vi "Test_PXF4_x2.vi"() -> ()   [LabVIEW 2019]
uses:
  <vilib>/NI/Modbus Library/API/Master/Modbus Master.lvclass
panel:
  in  "SV2_set":dbl=70.5 format="%.1f"
  in  "set_SV2":bool
  out "Out_2":bool
  out "SV2":dbl format="%.1f"
  out "PV2":dbl format="%.1f"
  in  "UID2":u8=2
  out "Out_1":bool
  in  "hysteresis_set":i16=1
  in  "set_hyst":bool
  out "time":timestamp format="%<%H:%M:%S\n%Y/%m/%d>T"
  out "hysteresis_get":u16
  in  "get_hyst":bool
  in  "set_SV":bool
  in  "interval":i32=1000
  in  "stop":bool
  out "SV1":dbl format="%.1f"
  out "PV1":dbl format="%.1f"
  in  "SV_set":dbl=70.5 format="%.1f"
  out "error out":errorcluster
  in  "UID1":u8=1
  in  "VISA":refnum<visa-resource-name>="COM7"
  # "CH 1"
  # "CH 2"
  # "°F"
  # "°F"
  # "°F"
  # "°F"
  # "°F"
  # "°F"
  # "°F"
  # "°F"
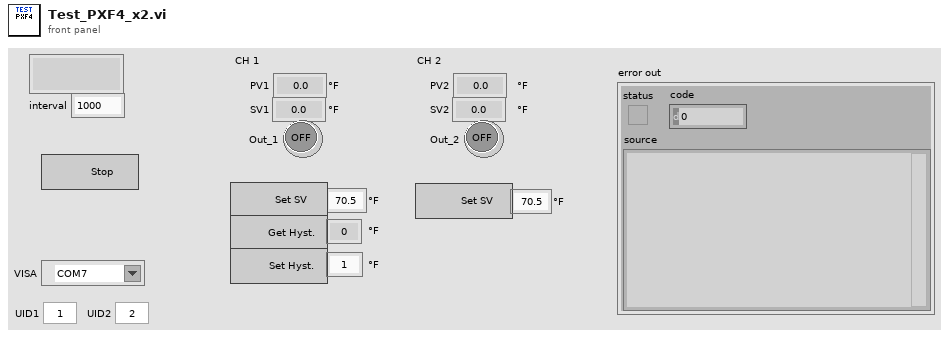
[diagram p1: front panel]
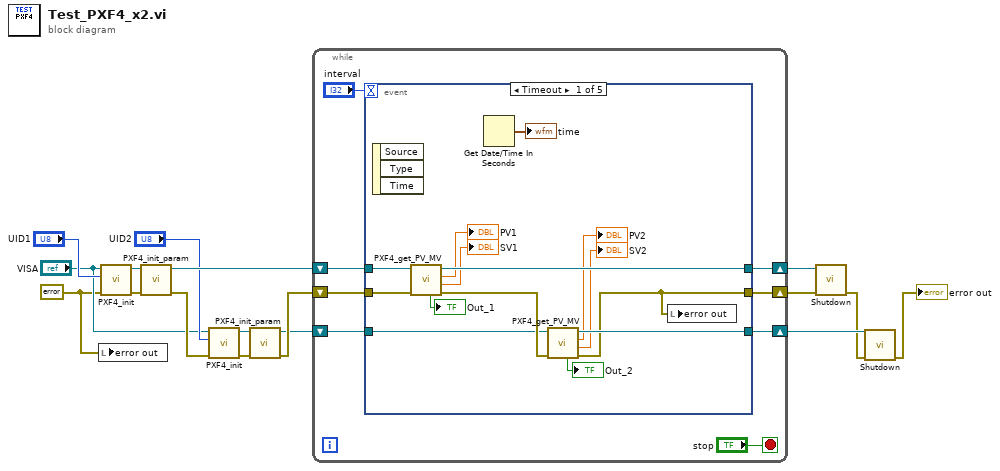
[diagram p0: block diagram]
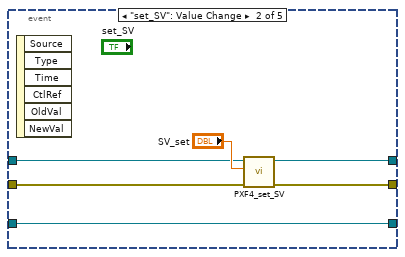
[diagram p2: hidden frame]
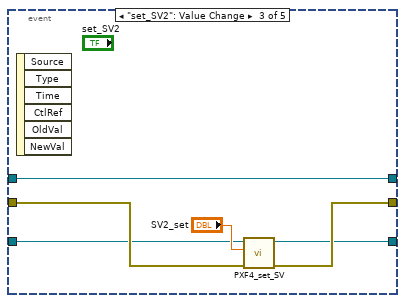
[diagram p3: hidden frame]
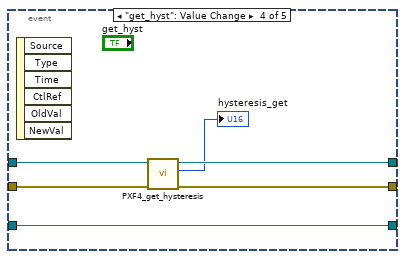
[diagram p4: hidden frame]
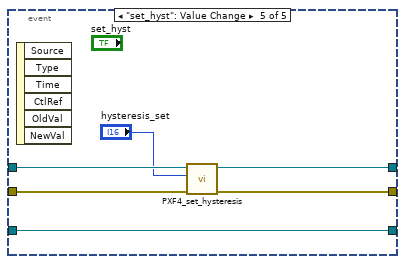
[diagram p5: hidden frame]
diagram:
  w1 = errorcluster {"status"=FALSE, "code"=0, "source"=""} ("error in")
  n1 = local write "error out"(w1) -> ()
  n2 = call "PXF4_init.vi"("error in"=w1, "unit_ID"="UID1", "VISA Refnum in"="VISA") -> ("error out"=w15:errorcluster, "Modbus Master out"=w16:refnum<class "Modbus Master.lvclass">)  [unwired: 7 in]
  n3 = call "PXF4_init_param.vi"("error in"=w15, "Modbus Master in"=w16) -> ("error out"=w9:errorcluster, "Modbus Master out"=w14:refnum<class "Modbus Master.lvclass">)  [unwired: 8 in]
  n4 = call "PXF4_init.vi"("error in"=w9, "unit_ID"="UID2", "VISA Refnum in"="VISA") -> ("error out"=w8:errorcluster, "Modbus Master out"=w11:refnum<class "Modbus Master.lvclass">)  [unwired: 7 in]
  n5 = call "PXF4_init_param.vi"("error in"=w8, "Modbus Master in"=w11) -> ("error out"=w7:errorcluster, "Modbus Master out"=w6:refnum<class "Modbus Master.lvclass">)  [unwired: 8 in]
  n6 = while {
    shift-right: [w22] -> w13
    shift-left: w14 -> [w25]
    shift-right: [w23] -> w12
    shift-left: w7 -> [w24]
    shift-right: [w18] -> w5
    shift-left: w6 -> [w19]
    stop <- "stop" stop-if-true
    n7 = event shown="[0] Timeout" {
      selector: _ -> [_ _ _ _ _]
      dyn-events: _ -> [_ _ _ _ _]
      timeout: "interval" -> [_ _ _ _ _]
      tunnel: w25 -> [w39 w41 w46 w57 w63]
      tunnel: w24 -> [w37 w42 w49 w56 w60]
      tunnel: [w26 w43 w50 w55 w61] -> w23
      tunnel: [w38 w44 w46 w54 w62] -> w22
      tunnel: w19 -> [w31 w40 w48 w52 w58]
      tunnel: [w30 w40 w47 w52 w58] -> w18
      event Timeout {
        n8 = event-data() -> ()  [unwired: 1 in, 3 out]
        n9 = call "PXF4_get_PV_MV.vi"("error in"=w37, "Modbus Master in"=w39) -> ("error out"=w32:errorcluster, "SV"=→"SV1":dbl, "PV"=→"PV1":dbl, "Modbus Master out"=w38:refnum<class "Modbus Master.lvclass">, "Output"=→"Out_1":bool)  [unwired: 5 in]
        n10 = Get Date/Time In Seconds() -> (seconds since 1Jan1904=→"time":timestamp)
        n11 = call "PXF4_get_PV_MV.vi"("error in"=w32, "Modbus Master in"=w31) -> ("error out"=w26:errorcluster, "SV"=→"SV2":dbl, "PV"=→"PV2":dbl, "Modbus Master out"=w30:refnum<class "Modbus Master.lvclass">, "Output"=→"Out_2":bool)  [unwired: 5 in]
        n12 = local write "error out"(w26) -> ()
      }
      event "set_SV": Value Change {
        n13 = event-data() -> ()  [unwired: 1 in, 6 out]
        n14 = call "PXF4_set_SV.vi"("error in"=w42, "SV"="SV_set", "Modbus Master in"=w41) -> ("error out"=w43:errorcluster, "Modbus Master out"=w44:refnum<class "Modbus Master.lvclass">)  [unwired: 7 in]
      }
      event "set_SV2": Value Change {
        n15 = event-data() -> ()  [unwired: 1 in, 6 out]
        n16 = call "PXF4_set_SV.vi"("error in"=w49, "SV"="SV2_set", "Modbus Master in"=w48) -> ("error out"=w50:errorcluster, "Modbus Master out"=w47:refnum<class "Modbus Master.lvclass">)  [unwired: 7 in]
      }
      event "get_hyst": Value Change {
        n17 = event-data() -> ()  [unwired: 1 in, 6 out]
        n18 = call "PXF4_get_hysteresis.vi"("error in"=w56, "Modbus Master in"=w57) -> ("error out"=w55:errorcluster, "hysteresis"=→"hysteresis_get":i16, "Modbus Master out"=w54:refnum<class "Modbus Master.lvclass">)  [unwired: 7 in]
      }
      event "set_hyst": Value Change {
        n19 = event-data() -> ()  [unwired: 1 in, 6 out]
        n20 = call "PXF4_set_hysteresis.vi"("error in"=w60, "hysteresis"="hysteresis_set", "Modbus Master in"=w63) -> ("error out"=w61:errorcluster, "Modbus Master out"=w62:refnum<class "Modbus Master.lvclass">)  [unwired: 7 in]
      }
    }
  }
  n21 = call-dynamic "Shutdown.vi"("error in"=w12, "Modbus master in"=w13) -> ("error out"=w4:errorcluster)  [unwired: 9 in]
  n22 = call-dynamic "Shutdown.vi"("error in"=w4, "Modbus master in"=w5) -> ("error out"=→"error out":errorcluster)  [unwired: 9 in]
